vi "预览报表-服务器版.vi"(11 "缓存数据路径":path=path "E:/Program Files (x86)/National Instruments/LabVIEW 2013/data/多点监测缓存数据文件-网络版/2016_10_23 00_23_16 #本机测试端口 #1.60 #1 #PC201410281258_8102.bin") -> ()   [LabVIEW 2013]
uses:
  <vilib>/event_ctls.llb/eventvkey.ctl
  <vilib>/Utility/NIReport.llb/HTML Report Image Alignment.ctl
  <vilib>/Utility/NIReport.llb/NI_report.lvclass
  <vilib>/Utility/NIReport.llb/Append Report Text (str wrap).vi
  <vilib>/Utility/NIReport.llb/NI_ReportGenerationCore.lvlib
panel:
  out "数值":string
  in  "删除文件":bool
  in  "保存":bool
  out "路径显示":path=path "C:/Users/Administrator/Desktop/35点监测报警信息报表模板 - 副本.doc"
  in  "取消":bool
  out "报警":string
  in  "生成报表":bool
  out "报警分析":i32(listbox)=-1
  in  "结论":string caption="结论（可编辑）"
  in  "附加信息":string caption="附加信息（可编辑）"
  out "探头信息":string
  out "探头地址":string
  out "实时曲线":cluster{"X":timestamp[], "Y":dbl[]}[](graph)
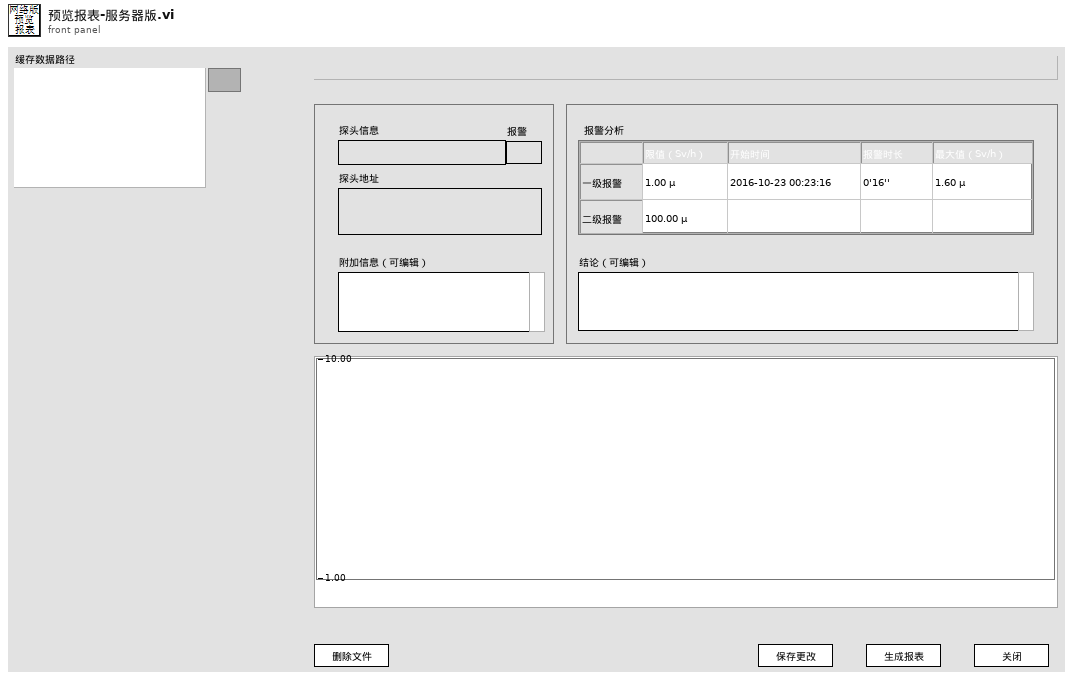
[diagram p1: front panel]
types:
  T1 = enum32{"Invalid", "Standard", "Closed", "Hidden", "Minimized", "Maximized"}
  T2 = typedef "eventvkey.ctl" = enum16{"ASCII", "Enter", "Return", "Shift", "Ctrl", "Alt", "Cmd", "Opt", "Caps", "NumLock", "Clear", "Break", "Up", "Down", "Left", "Right", "Insert", "Delete", "Home", "End", "PageUp", "PageDown", "Escape", "Help", "Pause", "ScrollLock", "F1", "F2", "F3", "F4", "F5", "F6", "F7", "F8", "F9", "F10", "F11", "F12", "F13", "F14", "F15", "F16", "F17", "F18", "F19", "F20", "F21", "F22", "F23", "F24", "Play", "VolumeUp", "VolumeDown", "Mute", "Two Byte Char"}
  T3 = cluster{"position (excel)":cluster{"row":i32, "column":i32}, "name (excel)":string, "bookmark (word)":string}
  T4 = enum16{"Standard Report", "HTML", "Word", "Excel"}
  T5 = enum16{"maximized", "minimized", "normal", "no change"}
  T6 = typedef "NI_ReportGenerationCore.lvlib/HTML Report Image Alignment.ctl" = enum16{"(default)", "LEFT", "RIGHT", "TOP", "TEXTTOP", "MIDDLE", "ABSMIDDLE", "BASELINE", "BOTTOM", "ABSBOTTOM"}
  T7 = cluster{"实时曲线":cluster{"X":timestamp[], "Y":dbl[]}[], "书签-键-值":string[][]}
  T8 = typedef "LVPoint32TypeDef.ctl" = cluster{"Horizontal":i32, "Vertical":i32}
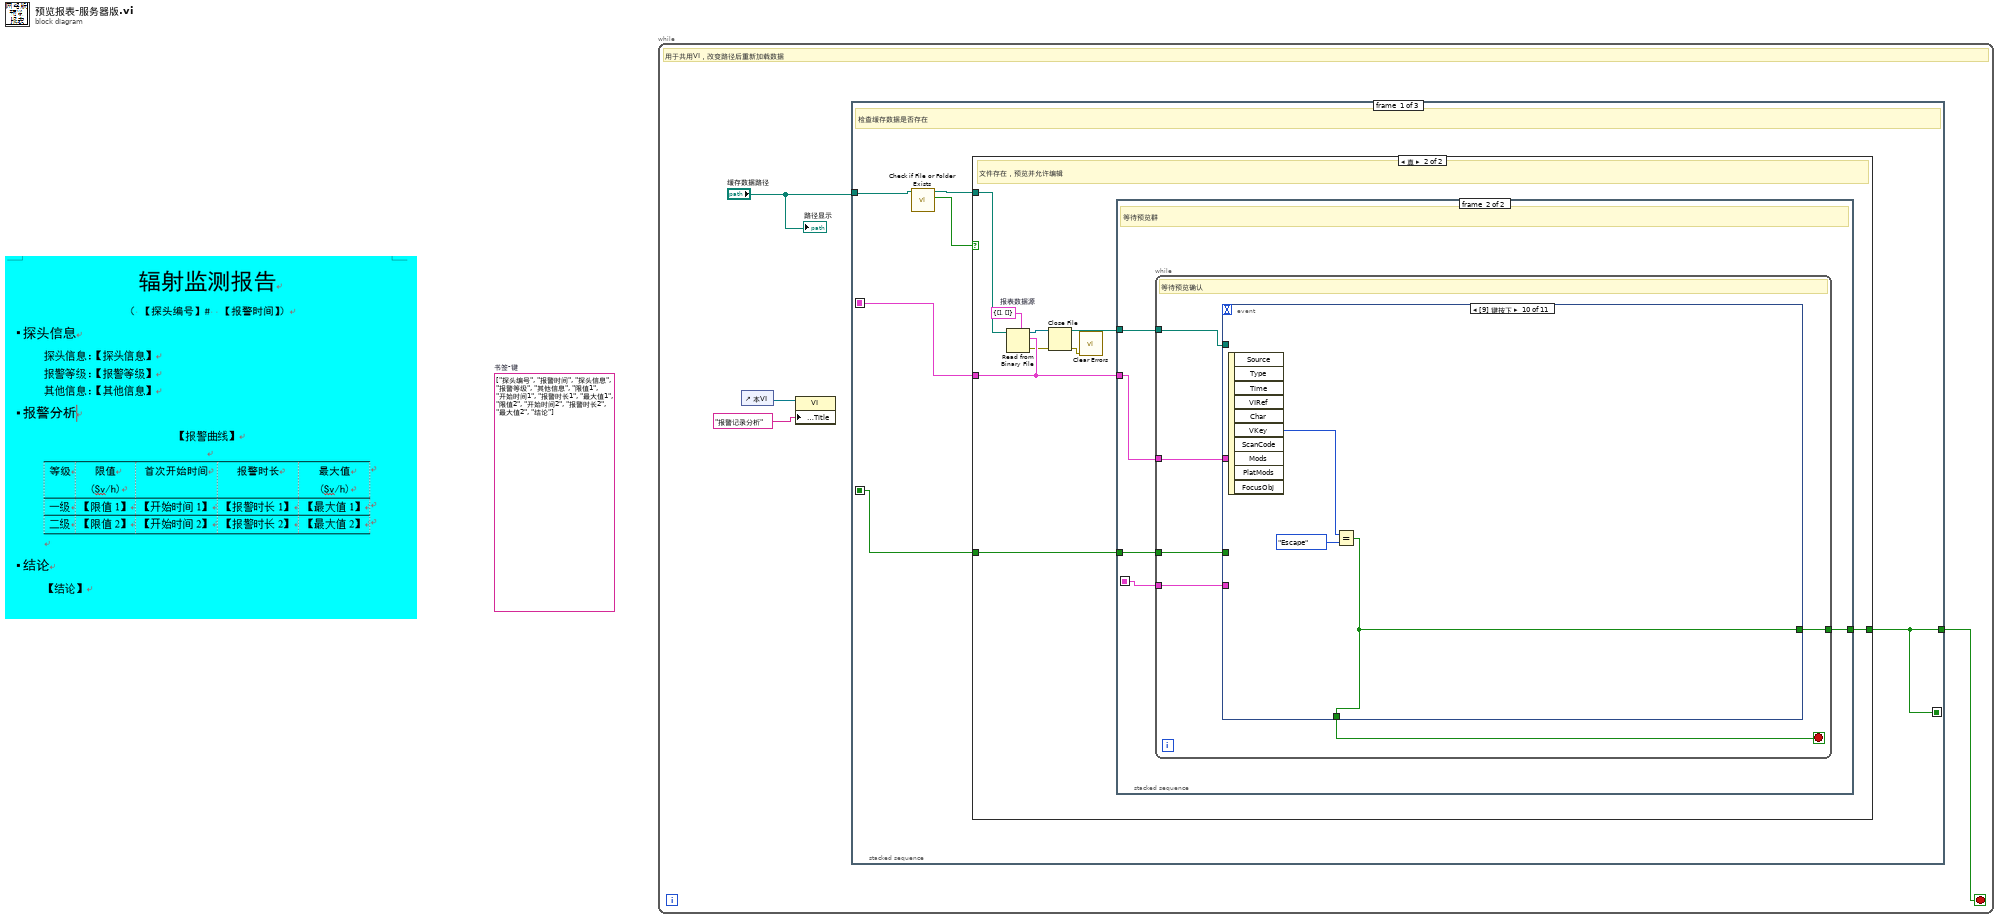
[diagram p0: block diagram]
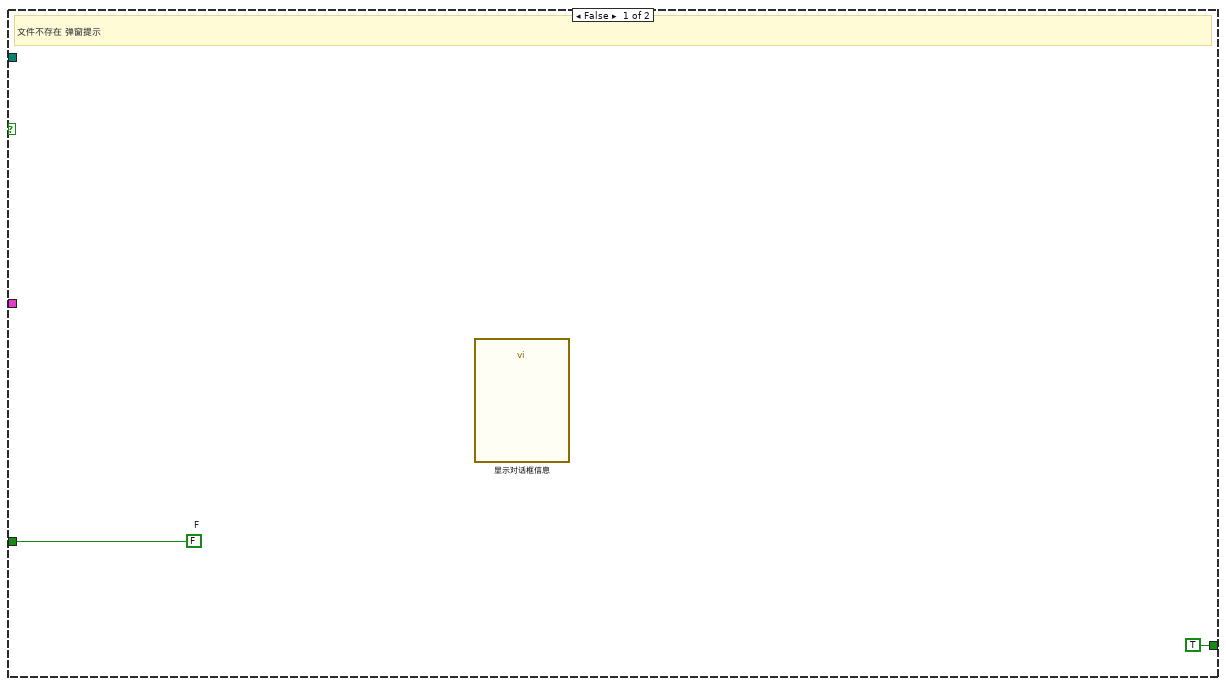
[diagram p2: hidden frame]
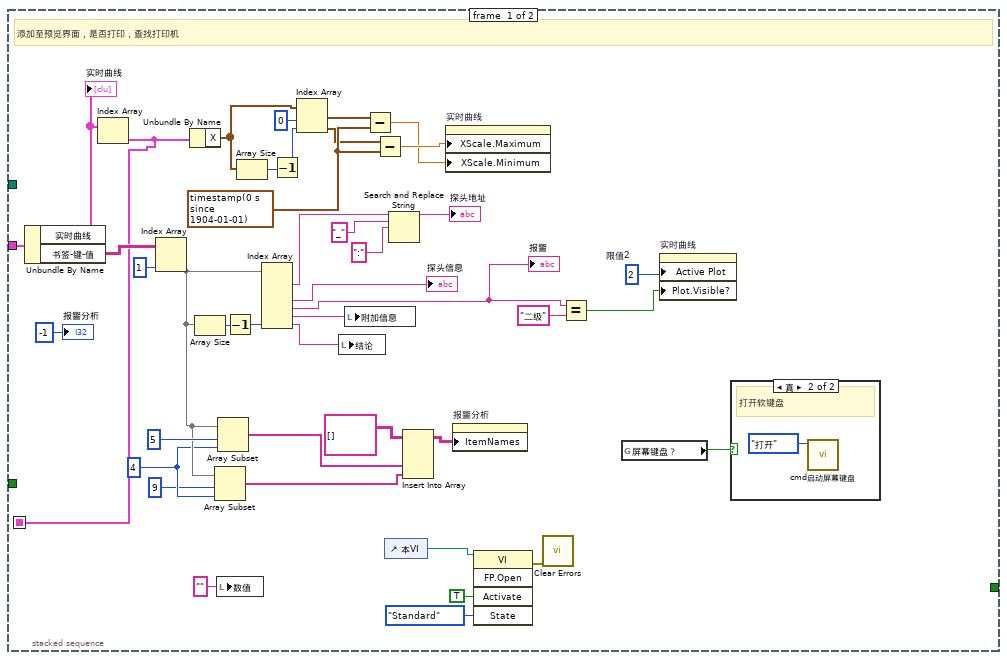
[diagram p3: hidden frame]
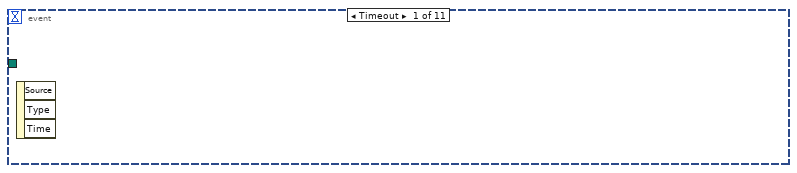
[diagram p5: hidden frame]
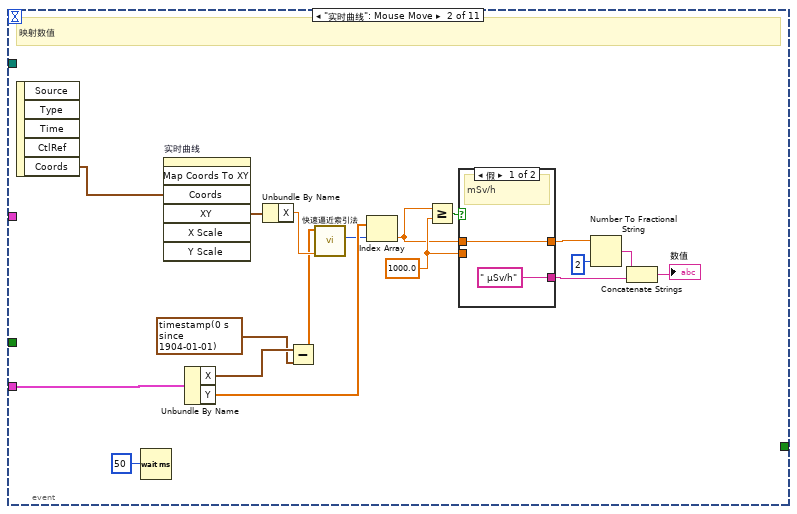
[diagram p6: hidden frame]
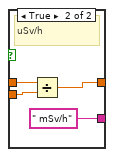
[diagram p7: hidden frame]
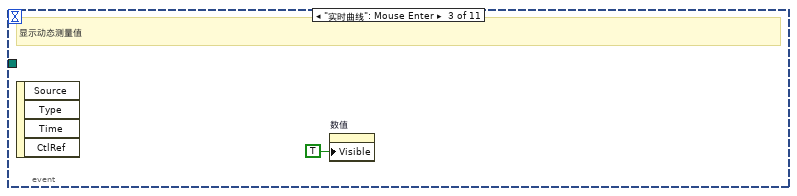
[diagram p8: hidden frame]
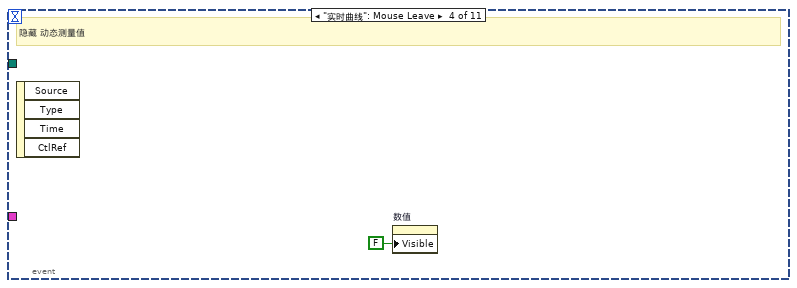
[diagram p9: hidden frame]
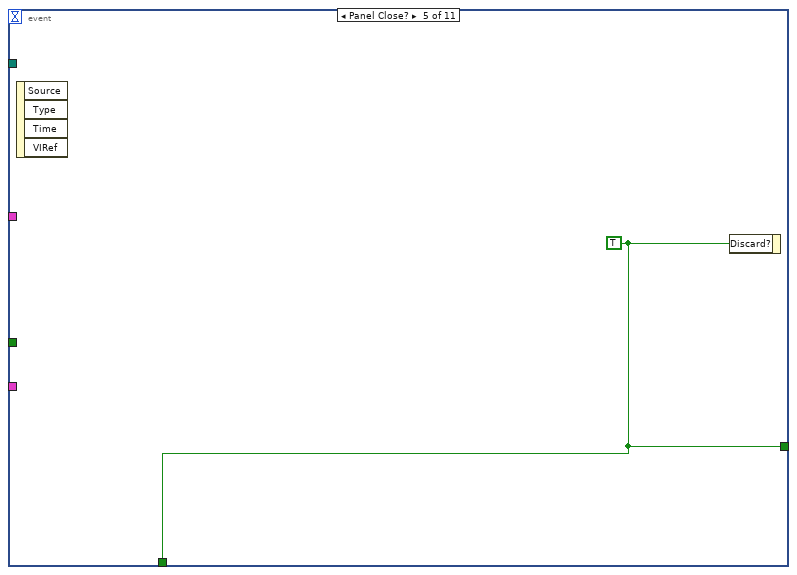
[diagram p10: hidden frame]
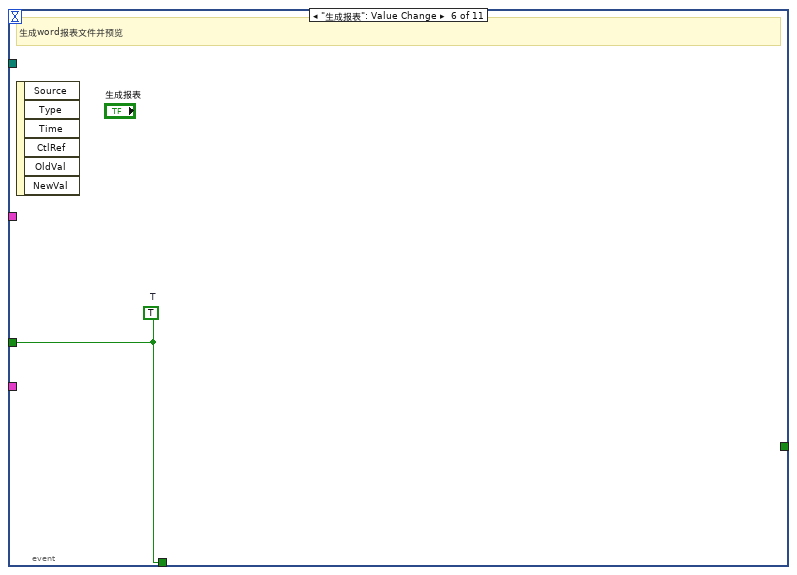
[diagram p11: hidden frame]
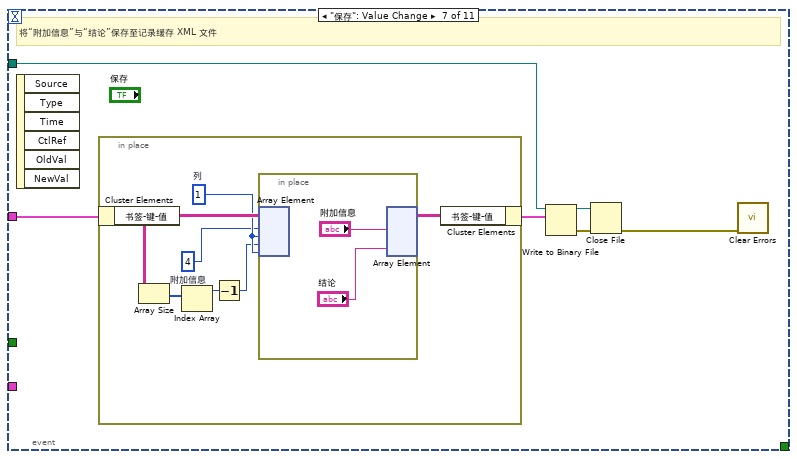
[diagram p12: hidden frame]
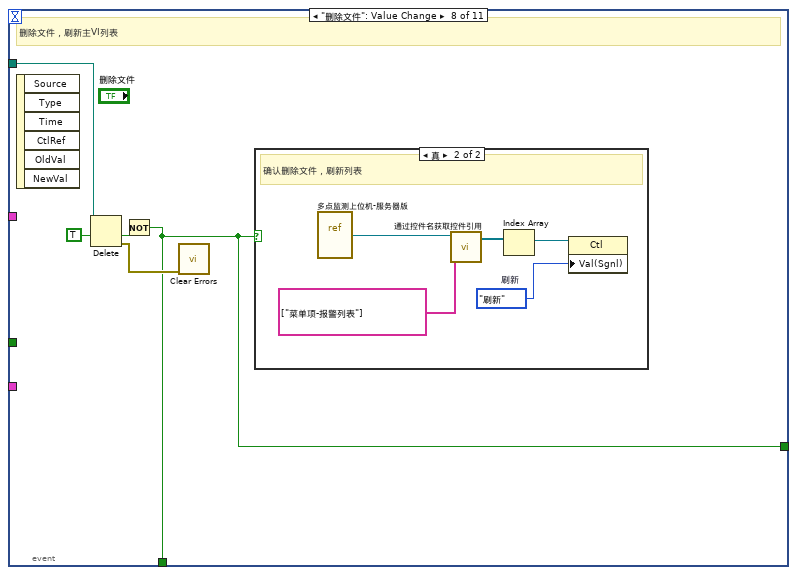
[diagram p13: hidden frame]
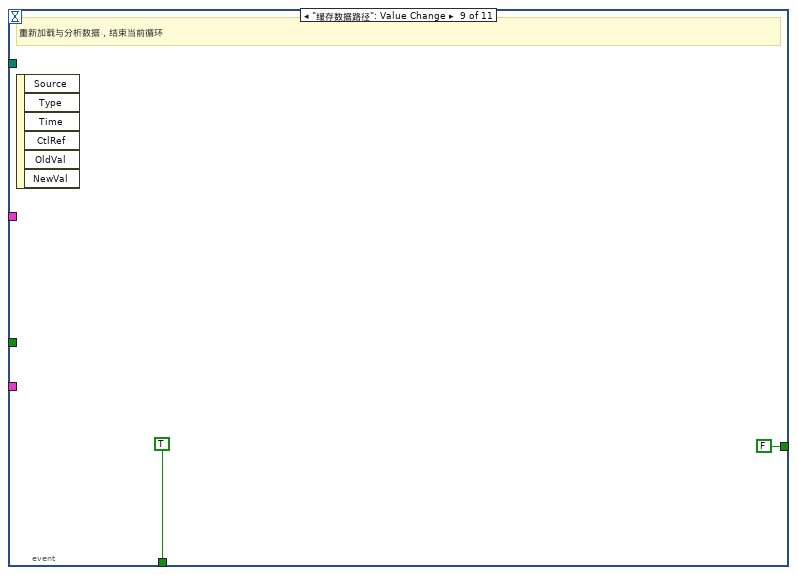
[diagram p15: hidden frame]
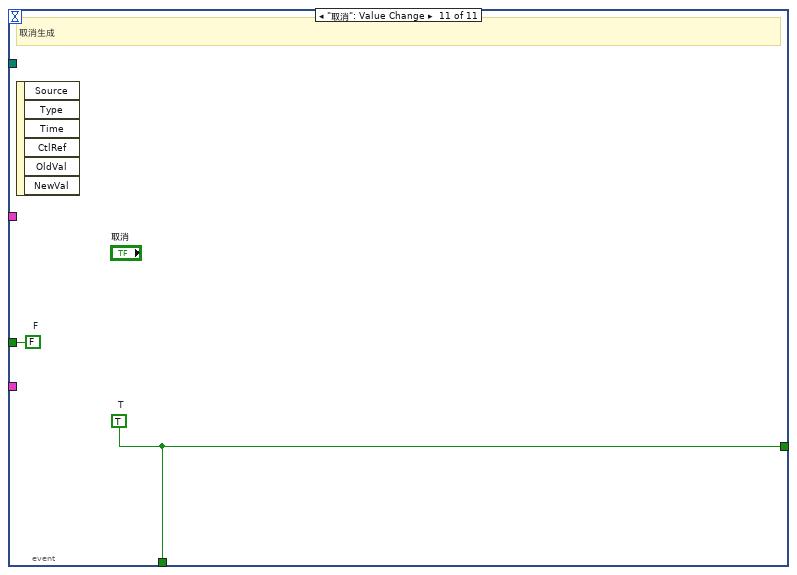
[diagram p16: hidden frame]
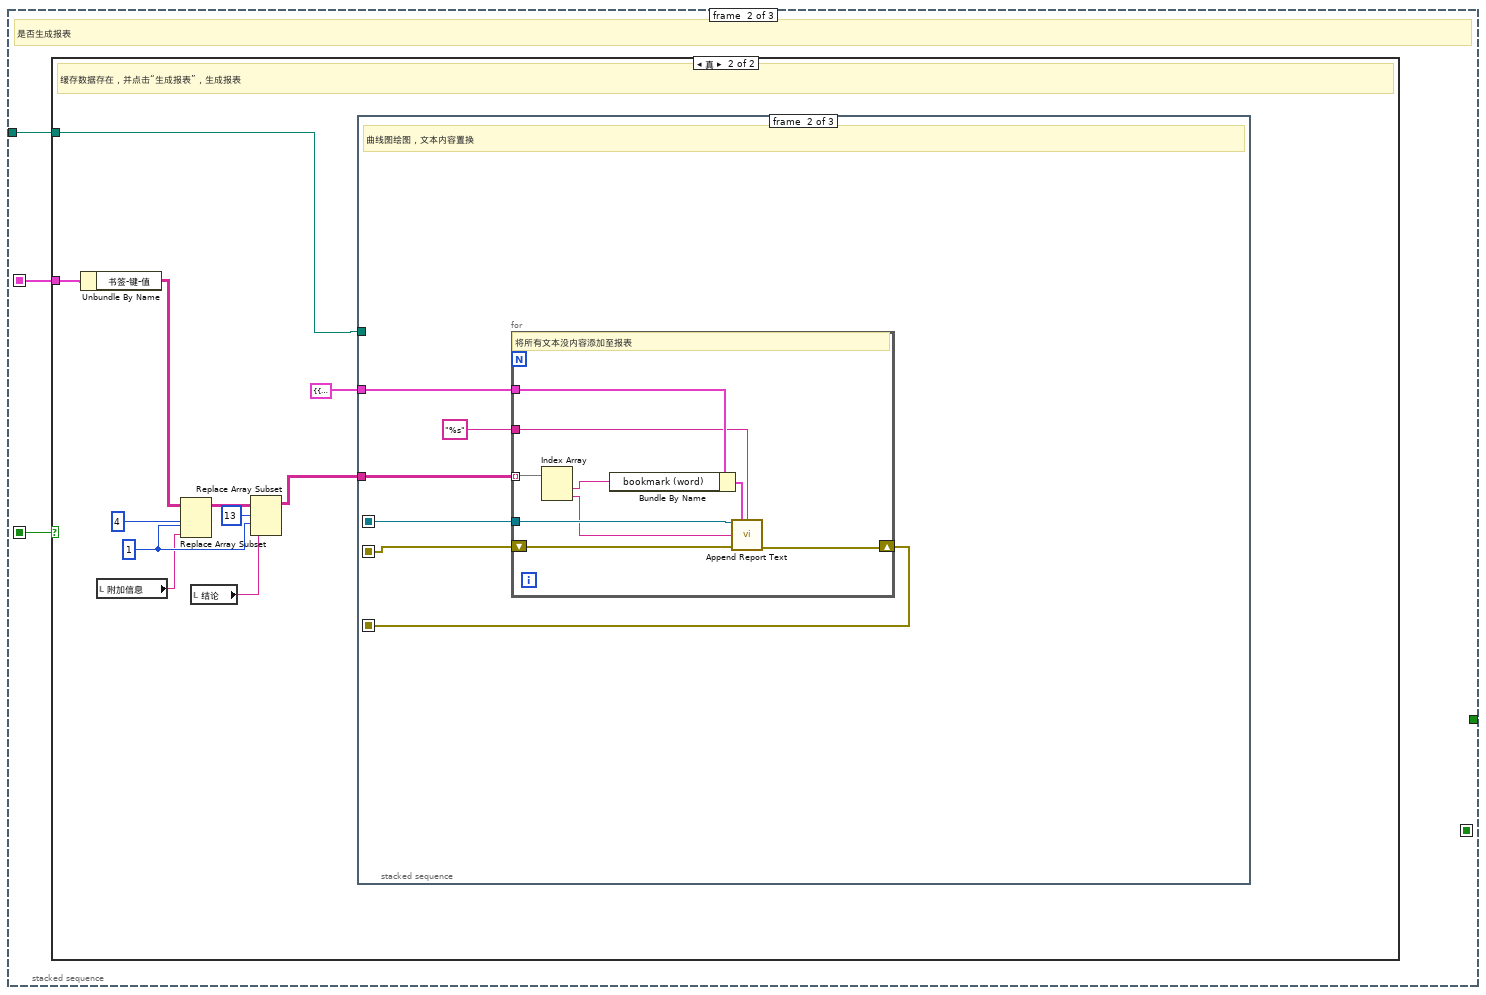
[diagram p17: hidden frame]
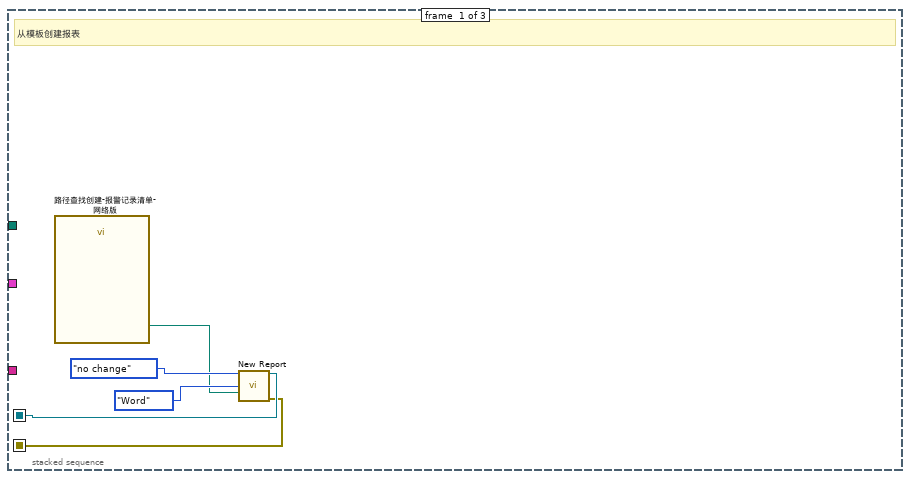
[diagram p19: hidden frame]
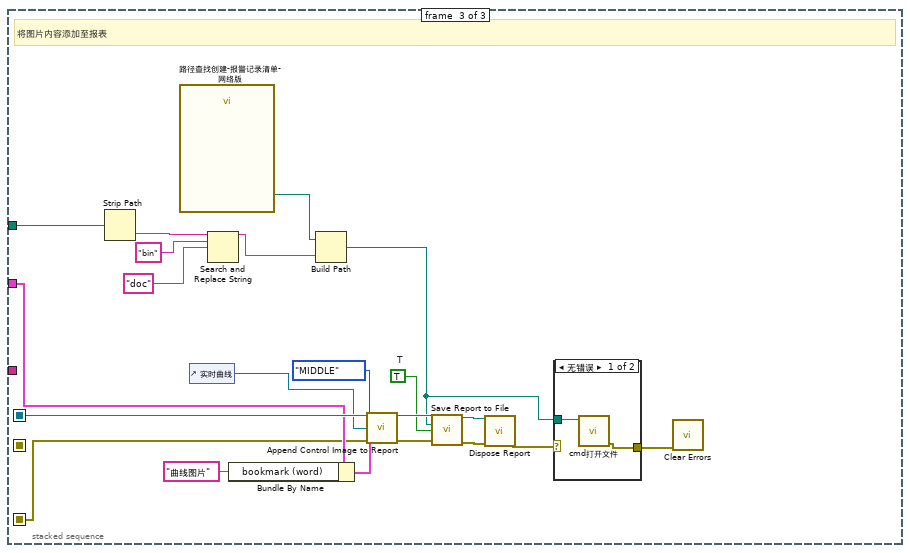
[diagram p20: hidden frame]
diagram:
  (unwired) string[] ["探头编号", "报警时间", "探头信息", "报警等级", "其他信息", "限值1", "开始时间1", "报警时长1", "最大值1", "限值2", "开始时间2", "报警时长2", "最大值2", "结论"]  # 书签-键
  n1 = while {
    stop <- w3 stop-if-true
    # "用于共用VI，改变路径后重新加载数据"
    n2 = control-ref of="本VI"() -> (w2:refnum<vi>)
    n3 = property class="VI"(reference=w2, "Front Panel.Title"="报警记录分析" ("前面板窗口:标题")) -> ()  [unwired: 1 in, 2 out]
    n4 = stacked-sequence {
      seq-local: [w10 _ _] -> [_ w138 _]
      seq-local: [w8 _ _] -> [_ w137 _]
      seq-local: [w9 _ _] -> [_ _ w194]
      tunnel: "缓存数据路径" -> [w6 w136 _]
      tunnel: [w9 _ _] -> w3
      frame #0 {
        # "检查缓存数据是否存在"
        n5 = call <vilib>:"Check if File or Folder Exists.vi"("path"=w6) -> ("file or folder exists?"=w7:bool, "dup path"=w5:path)  [unwired: 8 in, 1 out]
        n6 = case shown="真" w7 {
          tunnel: [_ w18] -> w8
          tunnel: [w12 w21] -> w10
          tunnel: w5 -> [_ w17]
          tunnel: [TRUE ("T") w20] -> w9
          frame False {
            w12 = FALSE  # F
            # "文件不存在 弹窗提示"
            n7 = call "显示对话框信息"() -> ()  [unwired: 10 in, 2 out]
          }
          frame True {
            w19 = T7 {"实时曲线"=[], "书签-键-值"=[]}  # 报表数据源
            # "文件存在，预览并允许编辑"
            n8 = Read from Binary File(5:w19, 11:w17) -> (0:w14:errorcluster, 2:w18:T7, 3:w16:refnum<file>)  [unwired: 4 in, 1 out]
            n9 = Close File(refnum=w16, error in=w14) -> (path=w15:path, error out=w13:errorcluster)
            n10 = call <vilib>:"Clear Errors.vi"("error in (no error)"=w13) -> ()  [unwired: 6 in, 1 out]
            n11 = stacked-sequence {
              seq-local: [w24 _] -> [_ w65]
              tunnel: w18 -> [w63 w68]
              tunnel: [_ w69] -> w21
              tunnel: w15 -> [_ w67]
              tunnel: [_ w66] -> w20
              frame #0 {
                w34 = timestamp(0 s since 1904-01-01) ("seconds since 1Jan1904")
                w41 = u32 2  # 限值2
                w54 = 4 ("索引")
                # "添加至预览界面，是否打印，查找打印机"
                n12 = Unbundle By Name(w63) -> ("实时曲线"=w25:cluster{"X":timestamp[], "Y":dbl[]}[], "书签-键-值"=w62:string[][])
                "实时曲线" <- w25
                n13 = Index Array(array=w25) -> (element=w24:cluster{"X":timestamp[], "Y":dbl[]})  [unwired: 1 in]
                n14 = Index Array(array=w62, index (col)=1 ("禁用的索引 (列)")) -> (element=w55:string[])  [unwired: 1 in]
                n15 = Unbundle By Name(w24) -> ("X"=w36:timestamp[])
                n16 = Array Size(array=w55) -> (size(s)=w58:i32)
                n17 = Array Subset(array=w55, index=9 ("索引"), length=w54) -> (w50:string[])
                n18 = local write "数值"("" ("数值")) -> ()
                n19 = Array Subset(array=w55, index=5 ("索引"), length=w54) -> (w52:string[])
                n20 = Decrement(x=w58) -> (x-1=w57:i32)
                n21 = Array Size(array=w36) -> (size(s)=w39:i32)
                n22 = Index Array(array=w55, index #6=w57) -> (element #1=w29:string, element #3=→"探头信息":string, element #4=w43:string, element #5=w59:string, element #6=w48:string)  [unwired: 5 in, 1 out]
                "报警" <- w43
                n23 = Decrement(x=w39) -> (x-1=w38:i32)
                n24 = Index Array(array=w36, index #1=0 ("索引"), index #2=w38) -> (element #1=w35:timestamp, element #2=w33:timestamp)
                n25 = local write "结论"(w48) -> ()
                n26 = local write "附加信息"(w59) -> ()
                n27 = Subtract(x=w35, y=w34) -> (x-y=w31:dbl)
                n28 = Subtract(x=w33, y=w34) -> (x-y=w32:dbl)
                n29 = control-ref of="本VI"() -> (w47:refnum<vi>)
                n30 = Search and Replace String(input string=w29, search string="_" ("搜索字符串"), replace string=":" ("搜索字符串")) -> (result string=→"探头地址":string)  [unwired: 5 in, 3 out]
                n31 = Insert Into Array(array=string[][] [] ("数组"), new element #1=w52, new element #2=w50) -> (w49:string[][])  [unwired: 2 in]
                n32 = property on="实时曲线" class="XYGraph (严格)"("XScale.Maximum"=w32, "XScale.Minimum"=w31) -> ()  [unwired: 2 in, 2 out]
                n33 = property on="报警分析" class="MCListbox (严格)"("ItemNames"=w49) -> ()  [unwired: 2 in, 2 out]
                n34 = invoke class="VI" method="FP.Open"(reference=w47, "Activate"=TRUE ("激活？"), "State"=T1."Standard" ("状态")) -> (error out=w44:errorcluster)  [unwired: 2 in, 4 out]
                n35 = call <vilib>:"Clear Errors.vi"("error in (no error)"=w44) -> ()  [unwired: 6 in, 1 out]
                n36 = Equal?(x=w43, y="二级") -> (x = y?=w40:bool)
                n37 = global read "全局变量-35点监测.vi" "屏幕键盘？"() -> (w22:bool)
                n38 = property on="实时曲线" class="XYGraph (严格)"("Active Plot"=w41, "Plot.Visible?"=w40) -> ()  [unwired: 2 in, 2 out]
                n39 = case shown="真" w22 {
                  frame False {
                  }
                  frame True {
                    # "打开软键盘"
                    n40 = call "cmd启动屏幕键盘.vi"("软键盘开关"=enum16{"关闭", "打开"}."打开") -> ()  [unwired: 10 in, 1 out]
                  }
                }
                "报警分析" <- -1 ("报警分析")
              }
              frame #1 {
                # "等待预览群"
                n41 = while {
                  tunnel: [w74] -> w69
                  tunnel: w68 -> [w73]
                  tunnel: w67 -> [w72]
                  tunnel: [w71] -> w66
                  tunnel: w65 -> [w70]
                  stop <- w75 stop-if-true
                  # "等待预览确认"
                  n42 = event shown="[9] 键按下" {
                    selector: _ -> [_ _ _ _ _ _ _ _ _ _ _]
                    dyn-events: _ -> [_ _ _ _ _ _ _ _ _ _ _]
                    timeout: _ -> [_ _ _ _ _ _ _ _ _ _ _]
                    tunnel: [_ _ _ _ w102 w103 _ w119 TRUE ("T") w131 w134] -> w75
                    tunnel: [_ _ _ _ _ w103 _ _ _ _ w135] -> w74
                    tunnel: w73 -> [_ _ _ _ _ _ w109 _ _ _ _]
                    tunnel: w72 -> [_ _ _ _ _ _ w108 w122 _ _ _]
                    tunnel: [_ _ _ _ w102 _ _ w119 FALSE ("T") w131 w134] -> w71
                    tunnel: w70 -> [_ w92 _ _ _ _ _ _ _ _ _]
                    event Timeout {
                      n43 = event-data() -> ()  [unwired: 1 in, 3 out]
                    }
                    event "实时曲线": Mouse Move {
                      w88 = 1000.0 ("y")
                      # "映射数值"
                      n44 = event-data() -> ("Coords"=w93:T8)  [unwired: 1 in, 4 out]
                      n45 = Wait (ms)(milliseconds to wait=u32 50 ("等待时间（毫秒）")) -> ()  [unwired: 1 out]
                      n46 = invoke on="实时曲线" class="XY图 (严格)" method="Map Coords To XY"("Coords"=w93) -> ("XY"=w90:cluster{"X":dbl, "Y":dbl})  [unwired: 6 in, 6 out]
                      n47 = Unbundle By Name(w92) -> ("X"=w81:timestamp[], "Y"=w78:dbl[])
                      n48 = Unbundle By Name(w90) -> ("X"=w82:dbl)
                      n49 = Subtract(x=w81, y=timestamp(0 s since 1904-01-01)) -> (x-y=w79:dbl[])
                      n50 = call "快速逼近索引法.vi"("数值"=w82, "数组"=w79) -> ("最近索引"=w77:i32)  [unwired: 9 in]
                      n51 = Index Array(array=w78, index=w77) -> (element=w76:dbl)
                      n52 = Greater Or Equal?(x=w76, y=w88) -> (x >= y?=w89:bool)
                      n53 = case shown="假" w89 {
                        tunnel: w76 -> [w95 w99]
                        tunnel: w88 -> [_ w98]
                        tunnel: [w95 w97] -> w86
                        tunnel: [" μSv/h" " mSv/h"] -> w84
                        frame False {
                          # "mSv/h"
                        }
                        frame True {
                          # "uSv/h"
                          n54 = Divide(x=w99, y=w98) -> (x/y=w97:dbl)
                        }
                      }
                      n55 = Number To Fractional String(number=w86, precision (6)=i16 2 ("精度(6)")) -> (F-format string=w85:string)  [unwired: 2 in]
                      n56 = Concatenate Strings(w85, w84) -> (→"数值":string)
                    }
                    event "实时曲线": Mouse Enter {
                      # "显示动态测量值"
                      n57 = event-data() -> ()  [unwired: 1 in, 4 out]
                      n58 = property on="数值" class="Str"("Visible"=TRUE ("可见")) -> ()  [unwired: 2 in, 2 out]
                    }
                    event "实时曲线": Mouse Leave {
                      # "隐藏 动态测量值"
                      n59 = event-data() -> ()  [unwired: 1 in, 4 out]
                      n60 = property on="数值" class="Str"("Visible"=FALSE ("可见")) -> ()  [unwired: 2 in, 2 out]
                    }
                    event Panel Close? {
                      w102 = TRUE ("放弃？")
                      n61 = event-data() -> ()  [unwired: 1 in, 4 out]
                      n62 = event-data("Discard?"=w102) -> ()  [unwired: 1 in, 1 out]
                    }
                    event "生成报表": Value Change {
                      w103 = TRUE  # T
                      # "生成word报表文件并预览"
                      n63 = event-data() -> ()  [unwired: 1 in, 6 out]
                    }
                    event "保存": Value Change {
                      # "将“附加信息”与“结论”保存至记录缓存 XML 文件"
                      n64 = event-data() -> ()  [unwired: 1 in, 6 out]
                      n65 = in-place {
                        w112 = 1  # 列
                        w111 = 4  # 附加信息
                        n66 = in-place-cluster #1(w109) -> ("书签-键-值"=w116:string[][])
                        n67 = Array Size(array=w116) -> (size(s)=w115:i32[])
                        n68 = Index Array(array=w115) -> (element=w114:i32)  [unwired: 1 in]
                        n69 = Decrement(x=w114) -> (x-1=w110:i32)
                        n70 = in-place {
                          n71 = in-place-array #2(w116, w111, w112, w110, w112) -> ()  [unwired: 2 out]
                          n72 = in-place-array #2("附加信息", "结论") -> (w113:string[][])  [unwired: 4 out]
                        }
                        n73 = in-place-cluster #1("书签-键-值"=w113) -> (w107:T7)
                      }
                      n74 = Write to Binary File(file (use dialog)=w108, data=w107) -> (refnum out=w106:refnum<file>, error out=w105:errorcluster)  [unwired: 4 in, 1 out]
                      n75 = Close File(refnum=w106, error in=w105) -> (error out=w104:errorcluster)  [unwired: 1 out]
                      n76 = call <vilib>:"Clear Errors.vi"("error in (no error)"=w104) -> ()  [unwired: 6 in, 1 out]
                    }
                    event "删除文件": Value Change {
                      # "删除文件，刷新主VI列表"
                      n77 = event-data() -> ()  [unwired: 1 in, 6 out]
                      n78 = Delete(path (use dialog)=w122, confirm (F)=TRUE ("确认(F)")) -> (cancelled=w120:bool, error out=w123:errorcluster)  [unwired: 3 in, 1 out]
                      n79 = Not(x=w120) -> (.not. x?=w119:bool)
                      n80 = call <vilib>:"Clear Errors.vi"("error in (no error)"=w123) -> ()  [unwired: 6 in, 1 out]
                      n81 = case shown="真" w119 {
                        frame False {
                          # "取消删除"
                        }
                        frame True {
                          w124 = enum16{"刷新", "预览并生成报表", "删除记录", "复制选中项至剪贴板"}."刷新"  # 刷新
                          # "确认删除文件，刷新列表"
                          n82 = vi-ref "多点监测上位机-服务器版.vi"() -> (w128:refnum<vi>)
                          n83 = call "通过控件名获取控件引用.vi"("控件名数组"=string[] ["菜单项-报警列表"], "VI引用"=w128) -> ("控件引用输出"=w126:refnum<vi>[])  [unwired: 7 in, 2 out]
                          n84 = Index Array(array=w126) -> (element=w125:refnum<vi>)  [unwired: 1 in]
                          n85 = property class="Ctl"(reference=w125, "Val(Sgnl)"=w124) -> ()  [unwired: 1 in, 2 out]
                        }
                      }
                    }
                    event "缓存数据路径": Value Change {
                      # "重新加载与分析数据，结束当前循环"
                      n86 = event-data() -> ()  [unwired: 1 in, 6 out]
                    }
                    event Key Down {
                      n87 = event-data() -> ("VKey"=w133:T2)  [unwired: 1 in, 9 out]
                      n88 = Equal?(x=w133, y=eventvkey."Escape") -> (x = y?=w131:bool)
                    }
                    event "取消": Value Change {
                      w135 = FALSE  # F
                      w134 = TRUE  # T
                      # "取消生成"
                      n89 = event-data() -> ()  [unwired: 1 in, 6 out]
                    }
                  }
                }
              }
            }
          }
        }
      }
      frame #1 {
        # "是否生成报表"
        n90 = case shown="真" w138 {
          tunnel: w137 -> [_ w149]
          tunnel: w136 -> [_ w147]
          frame False {
            # "缓存数据不存在，或点击“取消”"
          }
          frame True {
            w143 = 1 ("禁用的索引 (列)")
            # "缓存数据存在，并点击“生成报表”，生成报表"
            n91 = Unbundle By Name(w149) -> ("书签-键-值"=w146:string[][])
            n92 = local read "附加信息"() -> (w141:string)
            n93 = Replace Array Subset(array=w146, new element=w141, index (row)=4 ("禁用的索引 (行)"), index (col)=w143) -> (w144:string[][])
            n94 = local read "结论"() -> (w140:string)
            n95 = Replace Array Subset(array=w144, new element=w140, index (row)=13 ("禁用的索引 (行)"), index (col)=w143) -> (w139:string[][])
            n96 = stacked-sequence {
              seq-local: [w152 _ _] -> [_ w159 w188]
              seq-local: [_ w155 _] -> [_ _ w174]
              seq-local: [w150 _ _] -> [_ w156 _]
              tunnel: w139 -> [_ w160 _]
              tunnel: T3 {"position (excel)"={"row"=0, "column"=0}, "name (excel)"="", "bookmark (word)"=""} ("MS Office parameters") -> [_ w157 w186]
              tunnel: w147 -> [_ _ w183]
              frame #0 {
                # "从模板创建报表"
                n97 = call "路径查找创建-报警记录清单-网络版.vi"() -> ("报表模板"=w151:path)  [unwired: 1 in, 10 out]
                n98 = call <vilib>:"New Report.vi"("window state (normal)"=T5."no change", "report type"=T4."Word", "template (empty)"=w151) -> ("report out"=w152:refnum<class "NI_report.lvclass">, "error out"=w150:errorcluster)  [unwired: 11 in]
              }
              frame #1 {
                # "曲线图绘图，文本内容置换"
                n99 = for {
                  tunnel: w160 -> [w169] mode=indexing
                  tunnel: w157 -> [w168]
                  tunnel: w159 -> [w165]
                  tunnel: "%s" ("format string (%.3f)") -> [w163]
                  shift-right: [w162] -> w155
                  shift-left: w156 -> [w161]
                  # "将所有文本没内容添加至报表"
                  n100 = Index Array(array=w169) -> (element #1=w167:string, element #2=w164:string)  [unwired: 2 in]
                  n101 = Bundle By Name(cluster=w168, "bookmark (word)"=w167) -> (w166:T3)
                  n102 = call-poly <vilib>:"Append Report Text.vi"("report in"=w165, "MS Office parameters"=w166, "format string (%.3f)"=w163, "text"=w164, "error in (no error)"=w161) -> ("error out"=w162:errorcluster)  [unwired: 7 in, 3 out]
                }
              }
              frame #2 {
                w176 = TRUE  # T
                # "将图片内容添加至报表"
                n103 = Strip Path(path=w183) -> (name=w182:string)  [unwired: 1 out]
                n104 = call "路径查找创建-报警记录清单-网络版.vi"() -> ("报表文件夹"=w179:path)  [unwired: 1 in, 10 out]
                n105 = control-ref of="实时曲线"() -> (w185:refnum<vi>)
                n106 = Search and Replace String(input string=w182, search string="bin" ("搜索字符串"), replace string="doc" ("搜索字符串")) -> (result string=w178:string)  [unwired: 5 in, 3 out]
                n107 = Bundle By Name(cluster=w186, "bookmark (word)"="曲线图片") -> (w187:T3)
                n108 = Build Path(base path=w179, name or relative path=w178) -> (appended path=w171:path)
                n109 = call-dynamic "Append Control Image to Report.vi"("report in"=w188, "alignment (default)"=HTML_Report_Image_Alignment."MIDDLE", "ctrl reference"=w185, "error in (no error)"=w174, "MS Office parameters"=w187) -> ("report out"=w177:refnum<class "NI_report.lvclass">, "error out"=w175:errorcluster)  [unwired: 7 in, 2 out]
                n110 = call-dynamic "Save Report to File.vi"("report in"=w177, "report file path"=w171, "prompt to replace? (F)"=w176, "error in (no error)"=w175) -> ("report out"=w184:refnum<class "NI_report.lvclass">, "error out"=w173:errorcluster)  [unwired: 10 in]
                n111 = call-dynamic "Dispose Report.vi"("report in"=w184, "error in (no error)"=w173) -> ("error out"=w170:errorcluster)  [unwired: 13 in]
                n112 = case shown="无错误" w170 {
                  selector: w170 -> [_ w193]
                  tunnel: [w192 w193] -> w172
                  tunnel: w171 -> [w191 _]
                  frame No Error {
                    n113 = call "cmd打开文件.vi"("文件路径"=w191) -> ("error out"=w192:errorcluster)  [unwired: 10 in]
                  }
                  frame Error {
                  }
                }
                n114 = call <vilib>:"Clear Errors.vi"("error in (no error)"=w172) -> ()  [unwired: 6 in, 1 out]
              }
            }
          }
        }
      }
      frame #2 {
        # "退出关闭本VI"
        n115 = case shown="真" w194 {
          frame False {
          }
          frame True {
            # "结束程序？"
            n116 = control-ref of="本VI"() -> (w200:refnum<vi>)
            n117 = call "cmd启动屏幕键盘.vi"("软键盘开关"=enum16{"关闭", "打开"}."关闭") -> ("error out"=w195:errorcluster)  [unwired: 10 in]
            n118 = invoke class="VI" method="FP.Close"(reference=w200, error in=w195) -> (reference out=w199:refnum<vi>, error out=w198:errorcluster)  [unwired: 1 in, 1 out]
            n119 = invoke class="VI" method="Abort VI"(reference=w199, error in=w198) -> (error out=w197:errorcluster)  [unwired: 1 in, 2 out]
            n120 = call <vilib>:"Clear Errors.vi"("error in (no error)"=w197) -> ()  [unwired: 6 in, 1 out]
          }
        }
      }
    }
    "路径显示" <- "缓存数据路径"
  }
